vi "Shooter Coerce.vi"(10 "Hood Setpoint":dbl, 11 "Flywheel Setpoint":dbl) -> (2 "Coerced Hood":dbl, 3 "Coerced Flywheel":dbl)   [LabVIEW 2019]
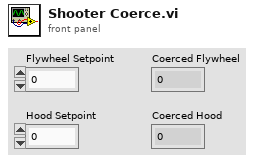
[diagram p1: front panel]
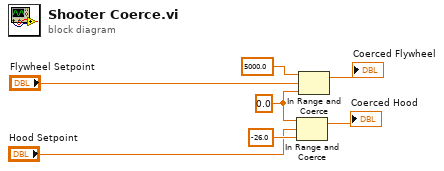
[diagram p0: block diagram]
diagram:
  w7 = 0.0 ("lower limit")
  n1 = In Range and Coerce(upper limit=w7, x="Hood Setpoint", lower limit=-26.0) -> (coerced(x)=→"Coerced Hood":dbl)  [unwired: 1 out]
  n2 = In Range and Coerce(upper limit=5000.0, x="Flywheel Setpoint", lower limit=w7) -> (coerced(x)=→"Coerced Flywheel":dbl)  [unwired: 1 out]
